vi "Climb_Globals.vi"() -> ()   [LabVIEW 2019]
uses:
  Subsystems/Climb/Climb_Pivot/Climb_Pivot_Cluster.ctl
  Subsystems/Climb/Climb_Pivot/Climb_Pivot_Control_States.ctl
  Subsystems/Climb/Climb_Elevator/Climb_Elevator_Cluster.ctl
  Subsystems/Climb/Climb_Elevator/Climb_Elevator_Control_States.ctl
  Subsystems/Climb/Climb_Transverse/Climb_Transverse_Cluster.ctl
  Subsystems/Climb/Climb_Transverse/Climb_Transverse_Control_States.ctl
panel:
  out "Pivot_At_Limit":bool
  in  "Climb_IMU":string="Climb_IMU"
  out "Pivot_Is_Moving":bool
  in  "Climb_Bottom_Limit":string="Climb_Bottom_Limit"
  in  "Climb_Top_Limit":string="Climb_Top_Limit"
  in  "Climb_Transverse_Execute_Notifier":refnum<notifier>
  in  "Climb_Transverse_Set_Notifier":refnum<notifier>
  in  "Climb_Elevator_Set_Notifier":refnum<notifier>
  in  "Climb_Elevator_Execute_Notifier":refnum<notifier>
  in  "Climb_Pivot_Execute_Notifier":refnum<notifier>
  in  "Climb_Pivot_Set_Notifier":refnum<notifier>
  in  "Climb_Transverse_Execute_Ref":string="Climb_Transverse_Execute_Ref"
  in  "Climb_Transverse_Set_Ref":string="Climb_Transverse_Set_Ref"
  in  "Climb_Elevator_Execute_Ref":string="Climb_Elevator_Execute_Ref"
  in  "Climb_Elevator_Set_Ref":string="Climb_Elevator_Set_Ref"
  in  "Climb_Pivot_Execute_Ref":string="Climb_Pivot_Execute_Ref"
  in  "Climb_Pivot_Set_Ref":string="Climb_Pivot_Set_Ref"
  in  "Climb_Transverse":string="Climb_Transverse"
  in  "Climb_Elevator_Left":string="Climb_Elevator_Left"
  in  "Climb_Elevator_Right":string="Climb_Elevator_Right"
  in  "Climb_Pivot":string="Climb_Pivot"
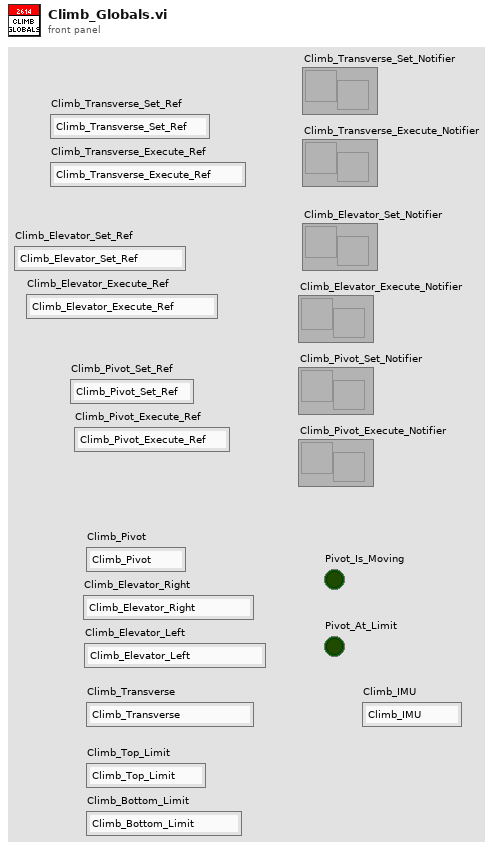
[diagram p1: front panel]
diagram:
